vi "Driver Config.vi"(5 "DriverID (\"\")":string, 7 "DriverType (\"\")":string, 8 "error in (no error)":errorcluster, 9 "port number (3363)":u16=3363, 10 "Configuration In (Empty)":string, 11 "TestStation Client (\"\")":string) -> (0 "error out":errorcluster, 1 "Serial Number":string, 2 "Configuration Out":string, 4 "LastCal":dbl, 6 "CalDue":dbl)   [LabVIEW 2011]
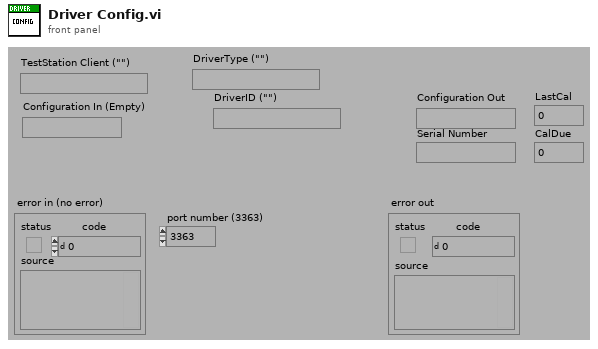
[diagram p1: front panel]
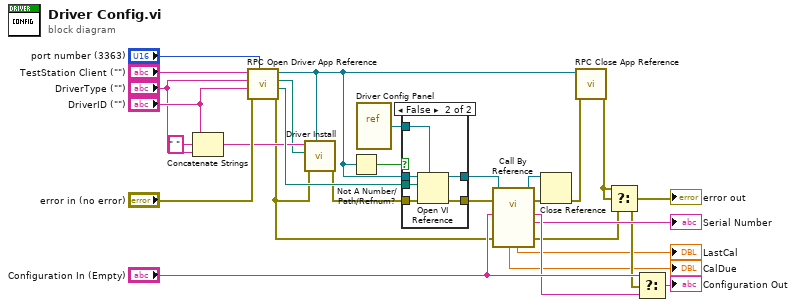
[diagram p0: block diagram]
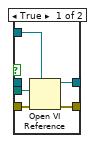
[diagram p2: hidden frame]
diagram:
  n1 = Concatenate Strings("DriverID (\"\")", " " ("string"), "DriverType (\"\")") -> (w5:string)
  n2 = call "RPC Open Driver App Reference.vi"("port number (3363)"="port number (3363)", "error in (no error)"="error in (no error)", "Driver ID (\"\")"="DriverID (\"\")", "Driver Type (\"\")"="DriverType (\"\")", "Client (\"\": open server reference)"="TestStation Client (\"\")") -> ("error out"=w3:errorcluster, "Driver Config Path"=w12:path, "Driver Component Path"=w4:path, "app reference"=w1:refnum<vi>)  [unwired: 3 out]
  n3 = call "Driver Install.vi"("app reference"=w1, "error in (no error)"=w3, "Driver Library Path"=w4, "DriverID DriverType (\"\")"=w5) -> ("error out"=w2:errorcluster)  [unwired: 7 out]
  n4 = Not A Number/Path/Refnum?(number/path/refnum=w1) -> (NaN/Path/Refnum?=w11:bool)
  n5 = vi-ref "Driver Config Panel.vi"() -> (w14:refnum<vi>)
  n6 = case shown="False" w11 {
    tunnel: [w33 w39] -> w15
    tunnel: w14 -> [w32 w38]
    tunnel: [w31 w37] -> w13
    tunnel: w12 -> [w30 w36]
    tunnel: w1 -> [_ w35]
    tunnel: w2 -> [w29 w34]
    frame True {
      n7 = Open VI Reference(type specifier VI Refnum (for type only)=w32, vi path=w30, error in (no error)=w29) -> (vi reference=w31:refnum<vi>, error out=w33:errorcluster)  [unwired: 3 out]
    }
    frame False {
      n8 = Open VI Reference(type specifier VI Refnum (for type only)=w38, application reference (local)=w35, vi path=w36, error in (no error)=w34) -> (vi reference=w37:refnum<vi>, error out=w39:errorcluster)  [unwired: 2 out]
    }
  }
  n9 = call-by-ref "?"(reference=w13, error in=w15, "error in (no error)"=w3, "Configuration In"="Configuration In (Empty)") -> (reference out=w27:refnum<vi>, error out=w28:errorcluster, 0:"error out"=w18:errorcluster, "Serial Number"=→"Serial Number":string, "Configuration Out"=w25:string, "LastCal"=→"LastCal":dbl, "CalDue"=→"CalDue":dbl)  [unwired: 5 in]
  n10 = Close Reference(reference=w27, error in (no error)=w28) -> (error out=w21:errorcluster)
  n11 = call "RPC Close App Reference.vi"("error in (no error)"=w21, "app reference"=w1) -> ("error out"=w19:errorcluster)  [unwired: 9 out]
  n12 = Select(t=w19, s=w19, f=w18) -> (s? t:f=w17:errorcluster)
  "error out" <- w17
  n13 = Select(t="Configuration In (Empty)", s=w17, f=w25) -> (s? t:f=→"Configuration Out":string)
